vi "SetPads1-64.vi"(9 "Y Channel":i32, 10 "Y Channels":cluster{"Label":string, "Pins":i32[]}[](array[cluster]), 11 "Pads 1-64":T1(array[cluster])) -> (3 "Pads 1-64":T1(array[cluster]))   [LabVIEW 2012, in "Virtual-PGA.lvlib"]
doc: "This VI links the Y input channels to pads."
uses:
  Virtual-PGA.lvlib
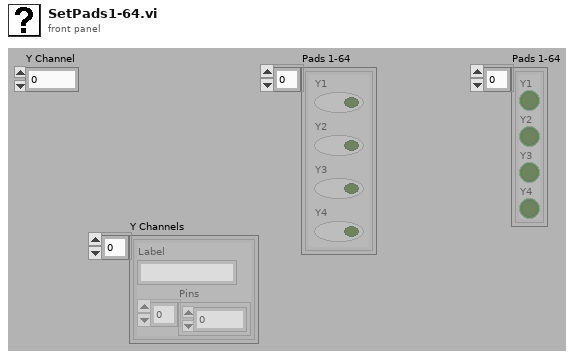
[diagram p1: front panel]
types:
  T1 = cluster{"Y1":bool, "Y2":bool, "Y3":bool, "Y4":bool}[]
  T2 = cluster{"Y1":bool, "Y2":bool, "Y3":bool, "Y4":bool}
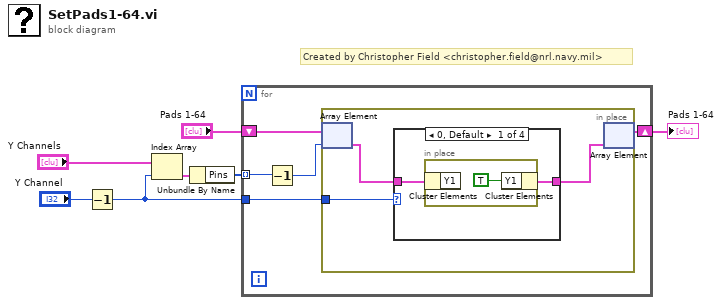
[diagram p0: block diagram]
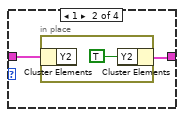
[diagram p2: hidden frame]
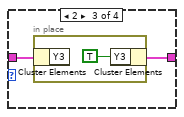
[diagram p3: hidden frame]
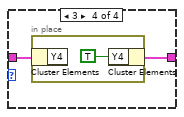
[diagram p4: hidden frame]
diagram:
  # "Created by Christopher Field <christopher.field@nrl.navy.mil>"
  n1 = Decrement(x="Y Channel") -> (x-1=w1:i32)
  n2 = Index Array(array="Y Channels", index=w1) -> (element=w6:cluster{"Label":string, "Pins":i32[]})
  n3 = Unbundle By Name(w6) -> ("Pins"=w5:i32[])
  n4 = for {
    tunnel: w5 -> [w12] mode=indexing
    tunnel: w1 -> [w8]
    shift-right: [w9] -> w3
    shift-left: "Pads 1-64" -> [w11]
    n5 = Decrement(x=w12) -> (x-1=w10:i32)
    n6 = in-place {
      in-place-border: w8 -> [w13]
      n7 = in-place-array #1(w11, w10) -> (w15:T2)
      n8 = case shown="0, Default" w13 {
        tunnel: w15 -> [w17 w20 w23 w26]
        tunnel: [w16 w19 w22 w25] -> w14
        frame 0, Default {
          n9 = in-place {
            n10 = in-place-cluster #2(w17) -> ()  [unwired: 1 out]
            n11 = in-place-cluster #2("Y1"=TRUE) -> (w16:T2)
          }
        }
        frame 1 {
          n12 = in-place {
            n13 = in-place-cluster #3(w20) -> ()  [unwired: 1 out]
            n14 = in-place-cluster #3("Y2"=TRUE) -> (w19:T2)
          }
        }
        frame 2 {
          n15 = in-place {
            n16 = in-place-cluster #4(w23) -> ()  [unwired: 1 out]
            n17 = in-place-cluster #4("Y3"=TRUE) -> (w22:T2)
          }
        }
        frame 3 {
          n18 = in-place {
            n19 = in-place-cluster #5(w26) -> ()  [unwired: 1 out]
            n20 = in-place-cluster #5("Y4"=TRUE) -> (w25:T2)
          }
        }
      }
      n21 = in-place-array #1(w14) -> (w9:T1)  [unwired: 1 out]
    }
  }
  "Pads 1-64" <- w3
